vi "SRV_PM_Add Packet to Queue.vi"(0 "Packet Data":u8[](array[numeric]) format="%.0x", 5 "New Packet Data":u8[](array[numeric]) format="%.0x") -> (8 "Array of Packets out":T1[](array[typedef]) {"Packet Data" format="%.0x"})   [LabVIEW 2009]
uses:
  SRV_PM_Packet.ctl
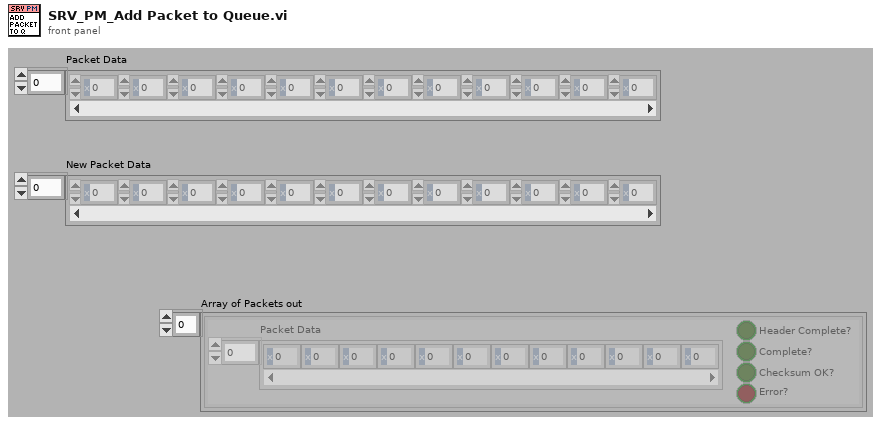
[diagram p1: front panel]
types:
  T1 = typedef "SRV_PM_Packet.ctl" = cluster{"Packet Data":u8[], "Header Complete?":bool, "Complete?":bool, "Checksum OK?":bool, "Error?":bool}
  T2 = typedef "SRV_PM_Packet.ctl" = cluster{"Packet Data":u8[], "Complete?":bool, "Error?":bool}
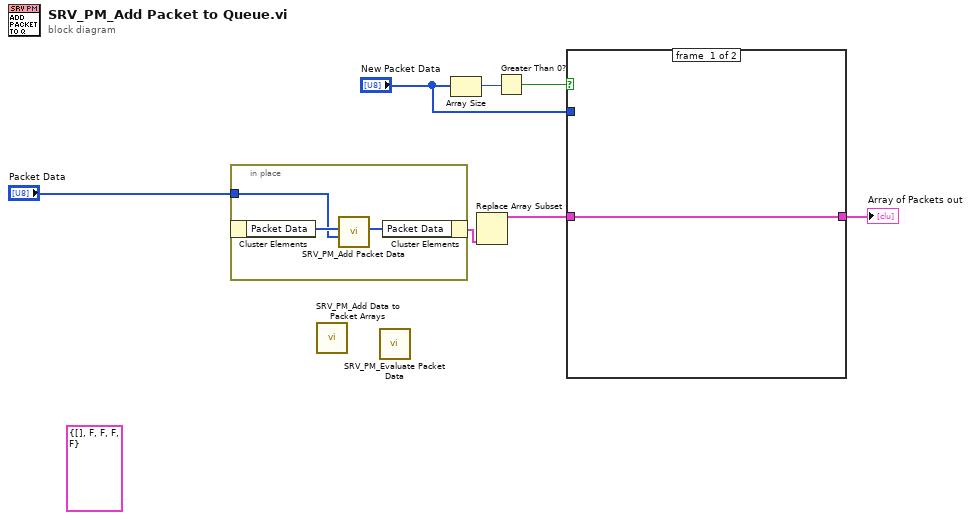
[diagram p0: block diagram]
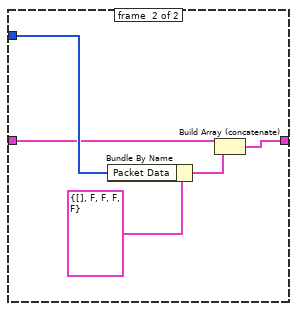
[diagram p2: hidden frame]
diagram:
  (unwired) T1 {"Packet Data"=[], "Header Complete?"=FALSE, "Complete?"=FALSE, "Checksum OK?"=FALSE, "Error?"=FALSE} ("Packet")
  n1 = in-place {
    in-place-border: "Packet Data" -> [w8]
    n2 = in-place-cluster #1() -> ("Packet Data"=w10:u8[])  [unwired: 1 in]
    n3 = call "SRV_PM_Add Packet Data.vi"("New Packet Data"=w8, "Packet Data"=w10) -> ("Packet Data out"=w9:u8[])  [unwired: 9 in]
    n4 = in-place-cluster #1("Packet Data"=w9) -> (w1:T2)
  }
  n5 = call "SRV_PM_Add Data to Packet Arrays.vi"() -> ()  [unwired: 15 in, 1 out]
  n6 = call "SRV_PM_Evaluate Packet Data.vi"() -> ()  [unwired: 11 in, 5 out]
  n7 = Array Size(array="New Packet Data") -> (size(s)=w6:i32)
  n8 = Replace Array Subset(new element=w1) -> (w4:T2[])  [unwired: 2 in]
  n9 = Greater Than 0?(x=w6) -> (x > 0?=w5:bool)
  n10 = case shown="True" w5 {
    tunnel: w4 -> [w11 w14]
    tunnel: [w11 w12] -> w3
    tunnel: "New Packet Data" -> [_ w15]
    frame #0 {
    }
    frame #1 {
      n11 = Bundle By Name(cluster=T1 {"Packet Data"=[], "Header Complete?"=FALSE, "Complete?"=FALSE, "Checksum OK?"=FALSE, "Error?"=FALSE} ("Packet"), "Packet Data"=w15) -> (w13:T1)
      n12 = Build Array (concatenate)(w14, w13) -> (w12:T2[])
    }
  }
  "Array of Packets out" <- w3
